vi "LOERN_BuildMenu.vi"(0 "XRef":T8, 1 "MenuRef":T7, 2 "Point":T5, 3 "Menu Type":T4, 4 "State In":T2={"Inputs"=1, "SelectedIndex"=0, "ClassInfo"=[]}) -> (14 "Fatal Error Out":T1)   [LabVIEW 2016, in "LV Object Event Registration Node.xnode"]
uses:
  LV Object Event Registration Node.xnode
  <vilib>/XNodeSupport/XNodeXNodeRef.ctl
  <vilib>/XNodeSupport/XNodeMenuRef.ctl
  <vilib>/XNodeSupport/XNodePoint.ctl
  <vilib>/XNodeSupport/XNodeInt.ctl
  <vilib>/XNodeSupport/XNodeMenuType.ctl
  LOERN_State.ctl
  LOERN_ClassInfo.ctl
  <vilib>/XNodeSupport/XNodeErrorCluster.ctl
  <vilib>/XNodeSupport/NI_XNodeSupport.lvlib
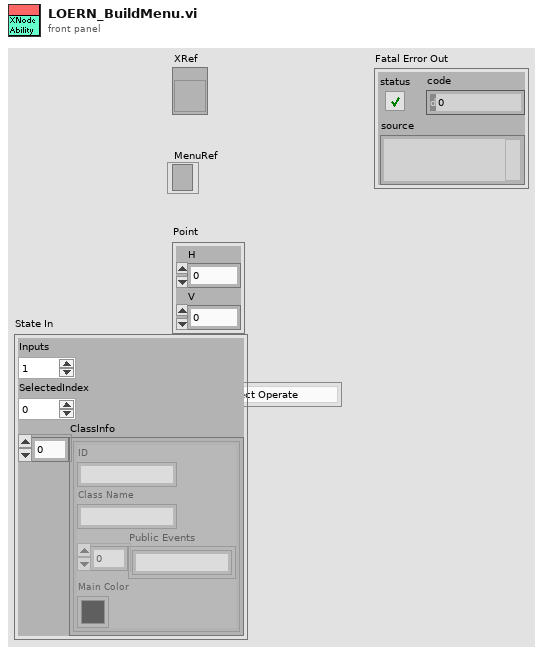
[diagram p1: front panel]
types:
  T1 = typedef "NI_XNodeSupport.lvlib/XNodeErrorCluster.ctl" = errorcluster
  T2 = typedef "LV Object Event Registration Node.xnode/LOERN_State.ctl" = cluster{"Inputs":u16, "SelectedIndex":i16, "ClassInfo":T3[]}
  T3 = typedef "LV Object Event Registration Node.xnode/LOERN_ClassInfo.ctl" = cluster{"ID":string, "Class Name":string, "Public Events":string[], "Main Color":u32}
  T4 = typedef "NI_XNodeSupport.lvlib/XNodeMenuType.ctl" = enum32{"Single Object Operate", "Single Object Popup", "Multi Object Popup Master", "Multi Object Popup Other"}
  T5 = typedef "NI_XNodeSupport.lvlib/XNodePoint.ctl" = cluster{"H":T6, "V":T6}
  T6 = typedef "NI_XNodeSupport.lvlib/XNodeInt.ctl" = i32
  T7 = typedef "NI_XNodeSupport.lvlib/XNodeMenuRef.ctl" = refnum<k9>
  T8 = typedef "NI_XNodeSupport.lvlib/XNodeXNodeRef.ctl" = refnum<vi>
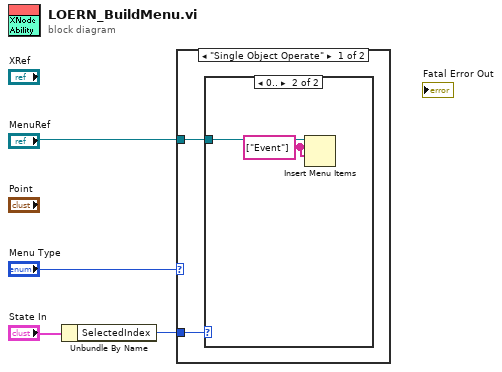
[diagram p0: block diagram]
diagram:
  n1 = Unbundle By Name("State In") -> ("SelectedIndex"=w2:i16)
  n2 = case shown="\"Single Object Operate\"" "Menu Type" {
    tunnel: w2 -> [w6 _]
    tunnel: "MenuRef" -> [w5 _]
    frame "Single Object Operate" {
      n3 = case shown="0.." w6 {
        tunnel: w5 -> [_ w8]
        frame Default {
        }
        frame 0.. {
          w7 = string[] ["Event"] ("item names")
          n4 = Insert Menu Items(7:w7, 8:w7, 9:w8) -> ()  [unwired: 3 in, 3 out]
        }
      }
    }
    frame "Single Object Popup", Default {
    }
  }
